vi "LVClass_WavefrontCorrectorSet WriteFile WavefrontCorrectorSetup.vi"(0 "WavefrontCorrectorSet in":refnum<class "WavefrontCorrectorSet.lvclass">, 11 "error in (no error)":errorcluster) -> (4 "WavefrontCorrectorSet out":refnum<class "WavefrontCorrectorSet.lvclass">, 15 "error out":errorcluster)   [LabVIEW 2020, in "WavefrontCorrectorSet.lvclass"]
uses:
  WavefrontCorrectorSet.lvclass
  WavefrontCorrectorSet.lvclass/WavefrontCorrectorSet.ctl
  <vilib>/Utility/xml.llb/Write to XML File(string).vi
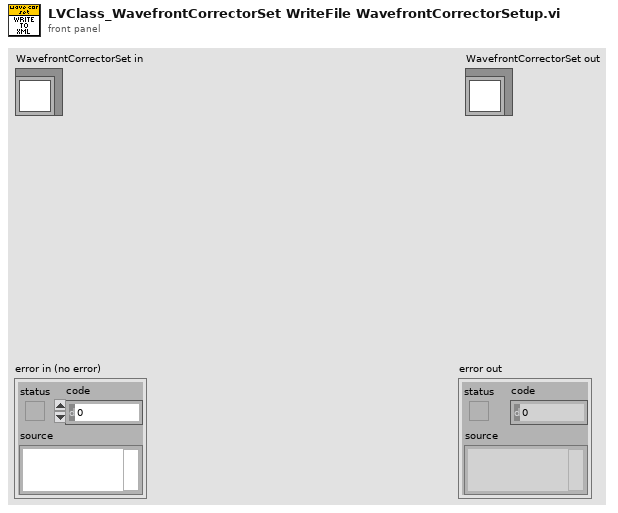
[diagram p1: front panel]
types:
  T1 = typedef "CameraParametersSetup.ctl" = cluster{"Name":string, "Type":T2, "Value":dbl, "BooleanValue":bool, "StringValue":string, "ConnectionParameter":bool}
  T2 = typedef "CameraParameters_Type.ctl" = enum16{"Integer", "Real", "String", "Boolean"}
  T3 = typedef "Wavefront Corrector states.ctl" = cluster{"Sleep after command apply_ms":i32, "Wavefront Corrector State":T4[], "WavefrontCorrectorOffsetState":sgl[]}
  T4 = typedef "Wavefront Corrector states - ONE.ctl" = cluster{"Max":sgl, "Min":sgl, "Validity":enum16{"valid", "fixed", "invalid"}, "Fixed_Position":sgl}
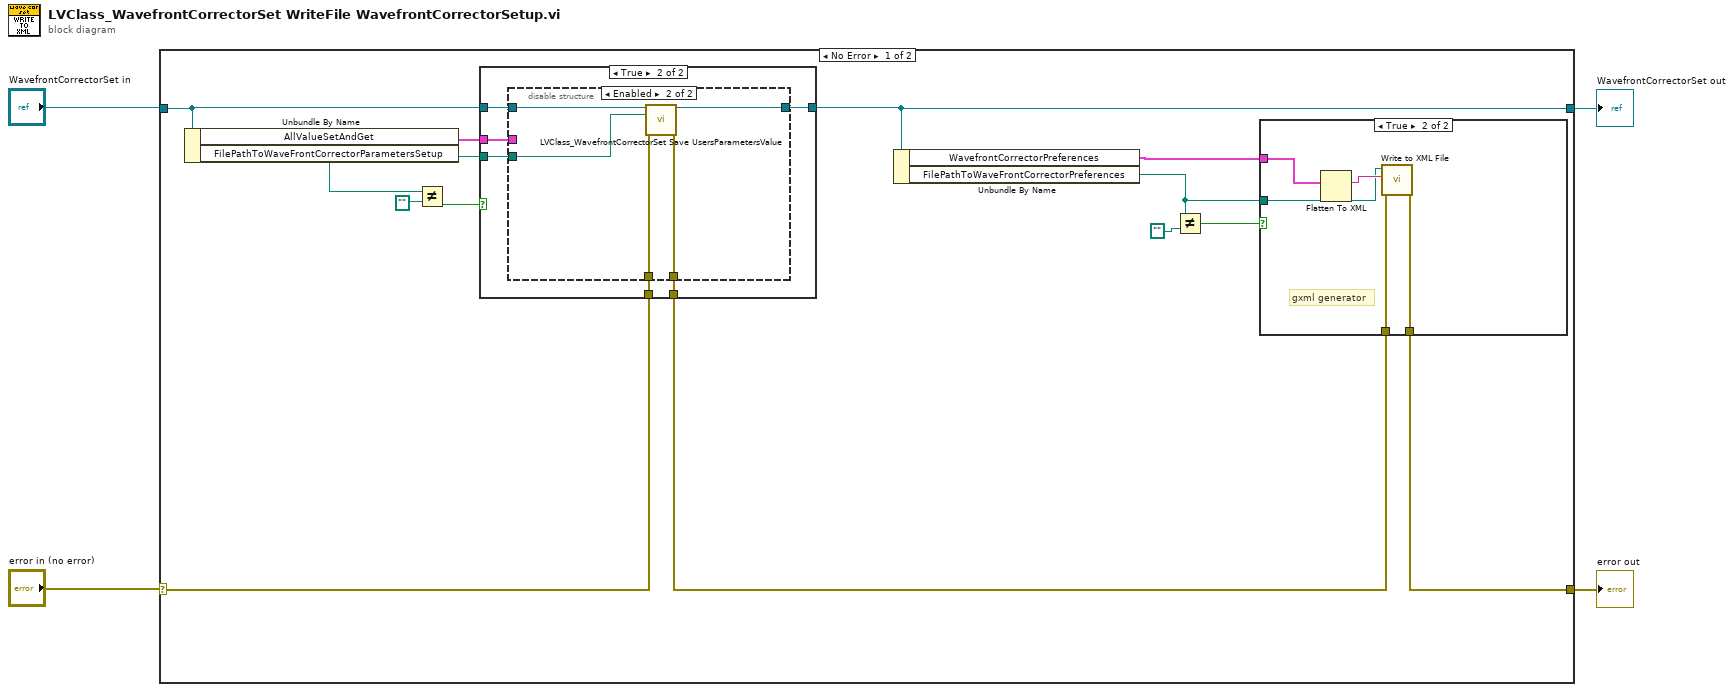
[diagram p0: block diagram]
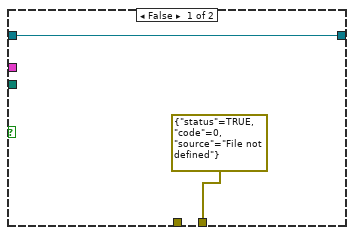
[diagram p2: hidden frame]
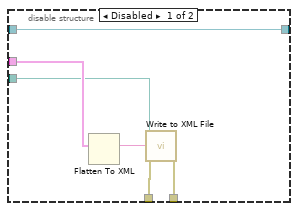
[diagram p3: hidden frame]
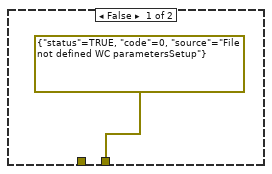
[diagram p4: hidden frame]
diagram:
  n1 = case shown="No Error" "error in (no error)" {
    selector: "error in (no error)" -> [w6 w44]
    tunnel: [w17 w44] -> w3
    tunnel: [w10 w43] -> w1
    tunnel: "WavefrontCorrectorSet in" -> [w11 w43]
    frame No Error {
      n2 = Unbundle By Name(w11) -> ("AllValueSetAndGet"=w12:T1[], "FilePathToWaveFrontCorrectorParametersSetup"=w8:path)
      n3 = Not Equal?(x=w8, y=path "") -> (x != y?=w7:bool)
      n4 = case shown="True" w7 {
        tunnel: w12 -> [_ w25]
        tunnel: w8 -> [_ w24]
        tunnel: w6 -> [_ w23]
        tunnel: [errorcluster {"status"=TRUE, "code"=0, "source"="File not defined"} ("error out") w22] -> w5
        tunnel: [w18 w21] -> w10
        tunnel: w11 -> [w18 w20]
        frame False {
        }
        frame True {
          n5 = disable-structure shown="Enabled" {
            disable-tunnel: w25 -> [w31 _]
            disable-tunnel: w24 -> [w29 w35]
            disable-tunnel: w23 -> [w28 w33]
            disable-tunnel: [w27 w32] -> w22
            disable-tunnel: w20 -> [w26 w36]
            disable-tunnel: [w26 w34] -> w21
            frame Disabled {
              n6 = Flatten To XML(6:w31) -> (2:w30:string)
              n7 = call-poly <vilib>:"Write to XML File.vi"("error in (no error)"=w28, "XML Input"=w30, "XML File Path"=w29) -> ("error out"=w27:errorcluster)  [unwired: 6 in, 2 out]
            }
            frame Enabled {
              n8 = call "LVClass_WavefrontCorrectorSet Save UsersParametersValue.vi"("WavefrontCorrectorSet in"=w36, "ParametersValue file path"=w35, "error in (no error)"=w33) -> ("WavefrontCorrectorSet out"=w34:refnum<class "WavefrontCorrectorSet.lvclass">, "error out"=w32:errorcluster)  [unwired: 11 in]
            }
          }
        }
      }
      n9 = Unbundle By Name(w10) -> ("WavefrontCorrectorPreferences"=w13:T3, "FilePathToWaveFrontCorrectorPreferences"=w14:path)
      n10 = Not Equal?(x=w14, y=path "") -> (x != y?=w15:bool)
      n11 = case shown="True" w15 {
        tunnel: w13 -> [_ w41]
        tunnel: w14 -> [_ w40]
        tunnel: w5 -> [_ w38]
        tunnel: [errorcluster {"status"=TRUE, "code"=0, "source"="File not defined WC parametersSetup"} ("error out") w39] -> w17
        frame False {
        }
        frame True {
          # "gxml generator"
          n12 = Flatten To XML(6:w41) -> (2:w42:string)
          n13 = call-poly <vilib>:"Write to XML File.vi"("error in (no error)"=w38, "XML Input"=w42, "XML File Path"=w40) -> ("error out"=w39:errorcluster)  [unwired: 6 in, 2 out]
        }
      }
    }
    frame Error {
    }
  }
  "error out" <- w3
  "WavefrontCorrectorSet out" <- w1
